vi "ReadCalibrationFilesSingle.vi"(8 "error in (no error)":errorcluster, 11 "MagSpecCamera in":refnum<class "MagSpecCamera.lvclass">) -> (0 "error out":errorcluster, 3 "MagSpecCamera in":refnum<class "MagSpecCamera.lvclass">)   [LabVIEW 2013, in "MagSpecCamera.lvclass"]
uses:
  MagSpecCamera.lvclass
  MagSpecCamera.lvclass/MagSpecCamera.ctl
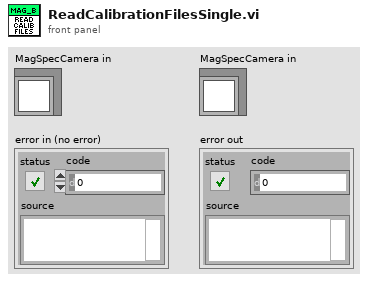
[diagram p1: front panel]
types:
  T1 = typedef "CalibrationCluster.ctl" = cluster{"bending angle Front":dbl[], "bending angle Side":dbl[], "screen [m] Front":dbl[], "screen [m] Side":dbl[], "momentum [MeV/c]":dbl[], "total path [m]":dbl[], "x[mm](rms)":dbl[], "x[mm](rms,b)":dbl[], "y[mm](rms)":dbl[], "y[mm](rms,b)":dbl[]}
  T2 = typedef "CameraSettings_File.ctl" = cluster{"FOV [mm]":dbl, "Left edge [mm]":dbl, "ROI Y offset":dbl, "ROI height":dbl, "ROI X offset":dbl, "ROI width":dbl, "Y center pixel":dbl, "Y Start":dbl, "Y End":dbl, "X Start":dbl, "X End":dbl, "rot [deg]":dbl}
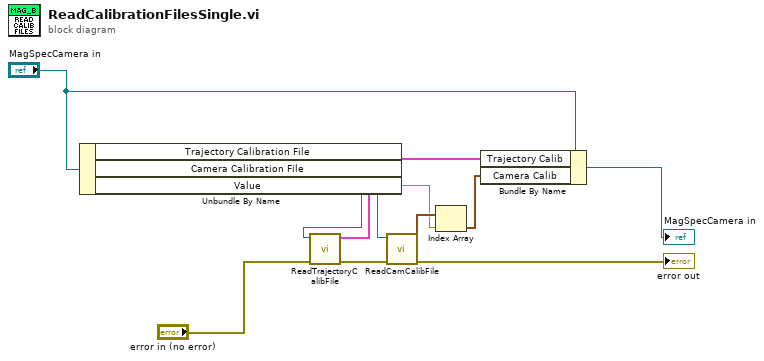
[diagram p0: block diagram]
diagram:
  n1 = Unbundle By Name("MagSpecCamera in") -> ("Trajectory Calibration File"=w4:path, "Camera Calibration File"=w7:path, "Value"=w1:dbl)
  n2 = call "ReadTrajectoryCalibFile.vi"("error in (no error)"="error in (no error)", "Spec_Calib_file in"=w4) -> ("error out"=w6:errorcluster, "Cluster"=w9:T1)  [unwired: 8 in]
  n3 = call "ReadCamCalibFile.vi"("error in (no error)"=w6, "Spec_Calib_file in"=w7) -> ("error out"=→"error out":errorcluster, "Cam Calib Array"=w3:T2[])  [unwired: 8 in]
  n4 = Index Array(array=w3, index=w1) -> (element=w2:T2)
  n5 = Bundle By Name(cluster="MagSpecCamera in", "Trajectory Calib"=w9, "Camera Calib"=w2) -> (→"MagSpecCamera in":refnum<class "MagSpecCamera.lvclass">)
